vi "Test Helper Loop Broadcast Stopping Twice Times Out.vi"(8 "error in (no error)":errorcluster, 11 "Helper Loop Test In":refnum<class "Helper Loop Test.lvclass">) -> (0 "error out":errorcluster, 3 "Helper Loop Test Out":refnum<class "Helper Loop Test.lvclass">)   [LabVIEW 2020, in "Helper Loop Test.lvclass"]
uses:
  Helper Loop Test.lvclass
  C:/Program Files (x86)/National Instruments/LabVIEW 2020/vi.lib/Astemes/LUnit/Test Case.lvclass
  source/Framework Test Suite/Mock Process/Mock Process.lvclass
  C:/Git/astemes-triarc-framework/source/Framework/Process/Process.lvclass
  <vilib>/Astemes/LUnit/Test Case.lvclass/Test Case.ctl
  <vilib>/Astemes/LUnit/LUnit Assertion Result.lvclass/LUnit Assertion Result.ctl
  <vilib>/Astemes/LUnit/LUnit Test Case Result.lvclass/LUnit Test Case Result.ctl
  <vilib>/Astemes/LUnit/LUnit Method Result.lvclass/LUnit Method Result.ctl
  source/Framework/Process/Process.lvclass/Process.ctl
  <vilib>/Astemes/LUnit/Set Assertion Type.vi
  <vilib>/Astemes/LUnit/Palette/Pass.vi
  <vilib>/Astemes/LUnit/Palette/Fail.vi
  source/Framework/Process/Private/SubVIs/Wait for finish.vi
  source/Framework/Process/Protected/Messaging/Enqueue Message.vi
  source/Framework/Process/Private/SubVIs/Set Lifecycle State.vi
  source/Framework/Process/Public/Lifecycle/Get Lifecycle State.vi
  <vilib>/Astemes/LUnit/LUnit Write Assertion Type.vi
  <vilib>/Astemes/LUnit/Add test result.vi
  <vilib>/Astemes/LUnit/LUnit Write Passed.vi
  <vilib>/Astemes/LUnit/LUnit Write Message.vi
  <vilib>/Astemes/LUnit/LUnit Write Description.vi
  source/Framework/Process/Private/SubVIs/Handle Debug Data.vi
  <vilib>/Utility/error.llb/Clear Errors.vi
  <vilib>/Astemes/LUnit/LUnit Record Assertion Result.vi
  source/Framework/Logging/Log Debug.vi
  <vilib>/AdvancedString/1D String Array to Delimited String.vi
  <vilib>/Utility/High Resolution Relative Seconds.vi
  <vilib>/Astemes/LUnit/LUnit Aggregate Assertion Results.vi
  <vilib>/Astemes/LUnit/Assertion Result/LUnit Read Status.vi
  <vilib>/Astemes/LUnit/LUnit Read Message.vi
  <vilib>/Astemes/LUnit/LUnit Read Description.vi
  <vilib>/Astemes/LUnit/Method Result/LUnit Merge Status.vi
  <vilib>/Astemes/LUnit/LUnit Concatenate result strings.vi
  <vilib>/Utility/error.llb/Error Cluster From Error Code.vi
  source/Framework/Process/Public/Read Name.vi
  <vilib>/Astemes/LUnit/LUnit Assertion Result.lvclass
  source/Framework/Process/Process.lvclass
  Helper Loop Test.lvclass/Helper Loop Test.ctl
  <vilib>/Astemes/LUnit/Test Case.lvclass
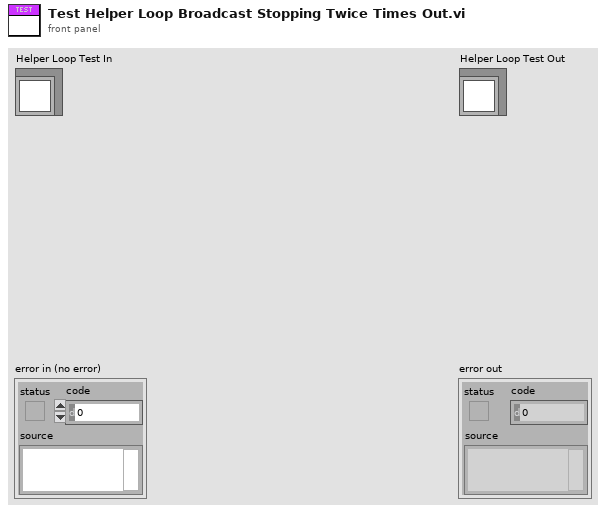
[diagram p1: front panel]
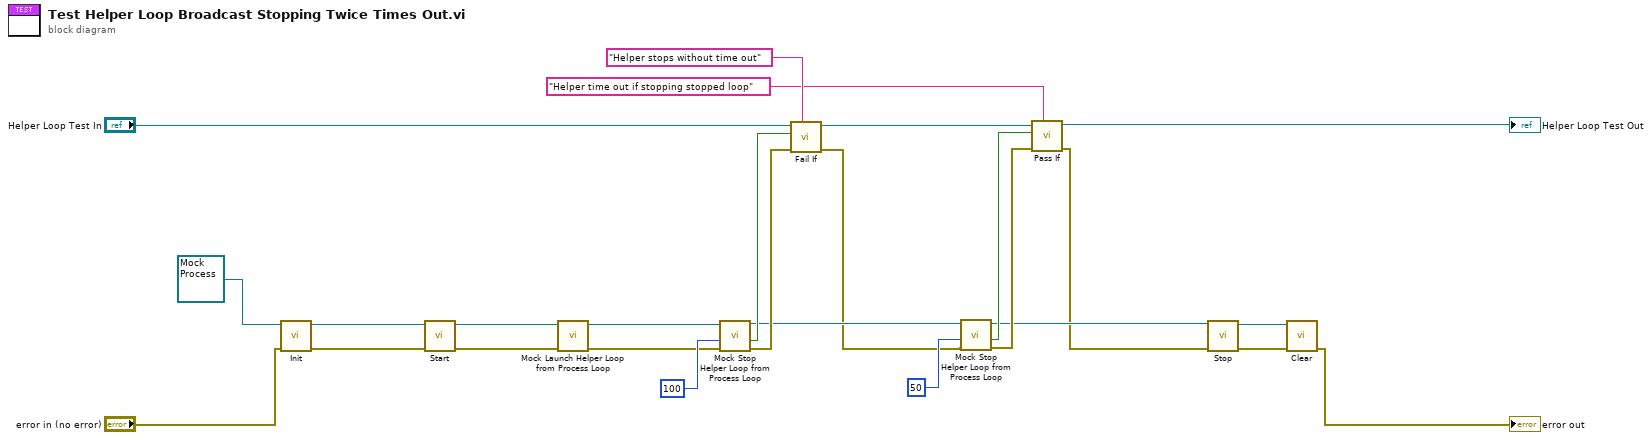
[diagram p0: block diagram]
diagram:
  n1 = call-dynamic "Init.vi"("error in (no error)"="error in (no error)", "Mock Process In"=refnum<class "Mock Process.lvclass"> refnum) -> ("error out"=w25:errorcluster, "Mock Process Out"=w26:refnum<class "Mock Process.lvclass">)  [unwired: 8 in]
  n2 = call "Start.vi"("error in (no error)"=w25, "Process In"=w26) -> ("error out"=w23:errorcluster, "Process Out"=w24:refnum<class "Mock Process.lvclass">)  [unwired: 7 in, 1 out]
  n3 = call "Mock Launch Helper Loop from Process Loop.vi"("error in (no error)"=w23, "Mock Process in"=w24) -> ("error out"=w12:errorcluster, "Mock Process out"=w13:refnum<class "Mock Process.lvclass">)  [unwired: 8 in]
  n4 = call "Mock Stop Helper Loop from Process Loop.vi"("error in (no error)"=w12, "timeout in ms (-1)"=100, "Mock Process in"=w13) -> ("error out"=w22:errorcluster, "timed out?"=w14:bool, "Mock Process out"=w7:refnum<class "Mock Process.lvclass">)  [unwired: 6 in]
  n5 = call <vilib>:"Fail If.vi"("Description"="Helper stops without time out", "error in (no error)"=w22, "Fail?"=w14, "LUnit Test Case In"="Helper Loop Test In") -> ("error out"=w6:errorcluster, "LUnit Test Case Out"=w3:refnum<class "Helper Loop Test.lvclass">)  [unwired: 6 in]
  n6 = call "Mock Stop Helper Loop from Process Loop.vi"("error in (no error)"=w6, "timeout in ms (-1)"=50, "Mock Process in"=w7) -> ("error out"=w8:errorcluster, "timed out?"=w11:bool, "Mock Process out"=w5:refnum<class "Mock Process.lvclass">)  [unwired: 6 in]
  n7 = call <vilib>:"Pass If.vi"("Description"="Helper time out if stopping stopped loop", "error in (no error)"=w8, "Pass?"=w11, "LUnit Test Case In"=w3) -> ("error out"=w4:errorcluster, "LUnit Test Case Out"=→"Helper Loop Test Out":refnum<class "Helper Loop Test.lvclass">)  [unwired: 6 in]
  n8 = call "Stop.vi"("error in (no error)"=w4, "Process In"=w5) -> ("error out"=w21:errorcluster, "Process Out"=w1:refnum<class "Mock Process.lvclass">)  [unwired: 7 in, 1 out]
  n9 = call-dynamic "Clear.vi"("error in (no error)"=w21, "Mock Process In"=w1) -> ("error out"=→"error out":errorcluster)  [unwired: 9 in]
